vi "Measurement.IVCurve.GetConfiguration.vi"(8 "error in (no error)":errorcluster, 11 "Measurement.IVCurve":refnum<class "Measurement.IVCurve.lvclass">) -> (0 "error out":errorcluster, 2 "Configuration":T1, 3 "Measurement.IVCurve out":refnum<class "Measurement.IVCurve.lvclass">)   [LabVIEW 2017, in "Measurement.IVCurve.lvclass"]
doc: "---------------------------------------------------------------\nJKI State Machine Objects™\nhttp://jki.net/state-machine-objects/\nCopyright (C) 2005-2015, JKI <info@jki.net>\nALL RIGHTS RESERVEDJKI State Machine Objects (SMO) 1.0.0.5\nJKI - JKI\nCopyright (c) 2016, JKI"
uses:
  Measurement.IVCurve.lvclass
  Typedefs/Configuration--Cluster.ctl
  Measurement/Typedefs/Measurement.Type--Enum.ctl
  Typedefs/Configuration.Hardware--Cluster.ctl
  Measurement/Typedefs/Configuration.SMU--Cluster.ctl
  SMU/Typedefs/Configuration--Cluster.ctl
  Typedefs/Configuration.Measurement--Cluster.ctl
  Measurement.IVCurve.lvclass/Measurement.IVCurve.ctl
  Measurement/Measurement.lvclass
  SMU/SMU.lvclass
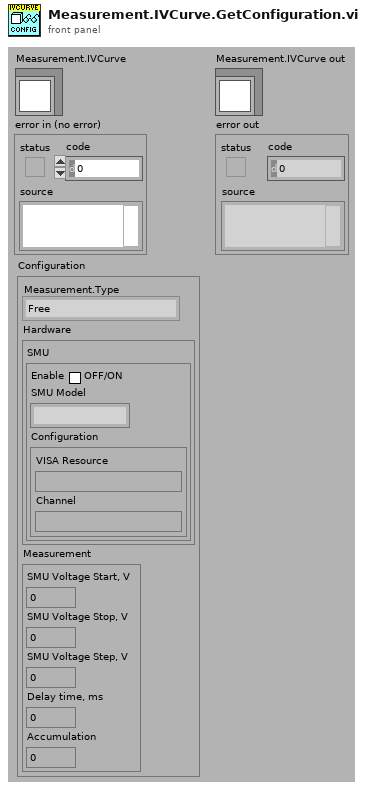
[diagram p1: front panel]
types:
  T1 = typedef "Measurement.IVCurve.lvclass/Configuration--Cluster.ctl" = cluster{"Measurement.Type":T2, "Hardware":T3, "Measurement":T6}
  T2 = typedef "Measurement.lvclass/Measurement.Type--Enum.ctl" = enum16{"Free", "I/V Curve", "Wavelength sweeping", "Photocurrent mapping"}
  T3 = typedef "Measurement.IVCurve.lvclass/Configuration.Hardware--Cluster.ctl" = cluster{"SMU":T4}
  T4 = typedef "Measurement.lvclass/Configuration.SMU--Cluster.ctl" = cluster{"Enable":bool, "SMU Model":string, "Configuration":T5}
  T5 = typedef "SMU.lvclass/Configuration--Cluster.ctl" = cluster{"VISA Resource":string, "Channel":string}
  T6 = typedef "Measurement.IVCurve.lvclass/Configuration.Measurement--Cluster.ctl" = cluster{"SMU Voltage Start, V":dbl, "SMU Voltage Stop, V":dbl, "SMU Voltage Step, V":dbl, "Delay time, ms":u16, "Accumulation":u16}
  T7 = typedef "Measurement.IVCurve.lvclass/PrivateData--Ref.ctl" = refnum<data-value>
  T8 = typedef "Measurement.IVCurve.lvclass/PrivateData--Cluster.ctl" = cluster{"Configuration":T1, "Dependencies":T9}
  T9 = typedef "Measurement.IVCurve.lvclass/Dependencies--Cluster.ctl" = cluster{"SMU":refnum<class "SMU.lvclass">}
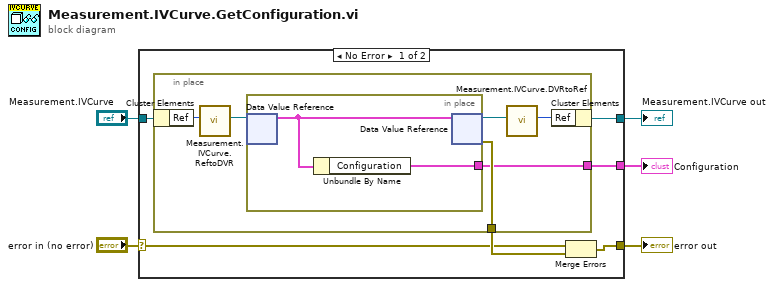
[diagram p0: block diagram]
diagram:
  n1 = case shown="No Error" "error in (no error)" {
    selector: "error in (no error)" -> [w7 w20]
    tunnel: "Measurement.IVCurve" -> [w8 w21]
    tunnel: [w9 w20] -> w4
    tunnel: [w11 w21] -> w3
    tunnel: [w6 _] -> w1
    frame No Error {
      n2 = in-place {
        in-place-border: [w17] -> w10
        in-place-border: [w12] -> w6
        n3 = in-place-cluster #1(w8) -> ("Ref"=w16:u32)
        n4 = call "Measurement.IVCurve.ReftoDVR.vi"("Ref"=w16) -> ("Ref"=w15:T7)  [unwired: 10 in]
        n5 = in-place {
          in-place-border: [w18] -> w12
          n6 = in-place-dvr #2(w15) -> (w19:T8)  [unwired: 1 out]
          n7 = Unbundle By Name(w19) -> ("Configuration"=w18:T1)
          n8 = in-place-dvr #2(w19) -> (w14:T7, w17:errorcluster)
        }
        n9 = call "Measurement.IVCurve.DVRtoRef.vi"("Ref"=w14) -> ("Ref"=w13:u32)  [unwired: 10 in]
        n10 = in-place-cluster #1("Ref"=w13) -> (w11:refnum<class "Measurement.IVCurve.lvclass">)
      }
      n11 = Merge Errors(w7, w10) -> (w9:errorcluster)
    }
    frame Error {
    }
  }
  "error out" <- w4
  "Measurement.IVCurve out" <- w3
  "Configuration" <- w1
